vi "sendEmail.vi"(6 "Queue limit":dbl=100.0, 7 "Mail":bool, 8 "error in (no error)":errorcluster, 9 "Recipient's Email Address Address":string="frouman@gmail.com", 10 "Queue Length":dbl, 11 "Acquisition in":refnum<class "Acquisition.lvclass">) -> (0 "error out":errorcluster, 3 "Acquisition out":refnum<class "Acquisition.lvclass">)   [LabVIEW 2014, in "Acquisition.lvclass"]
uses:
  Acquisition.lvclass
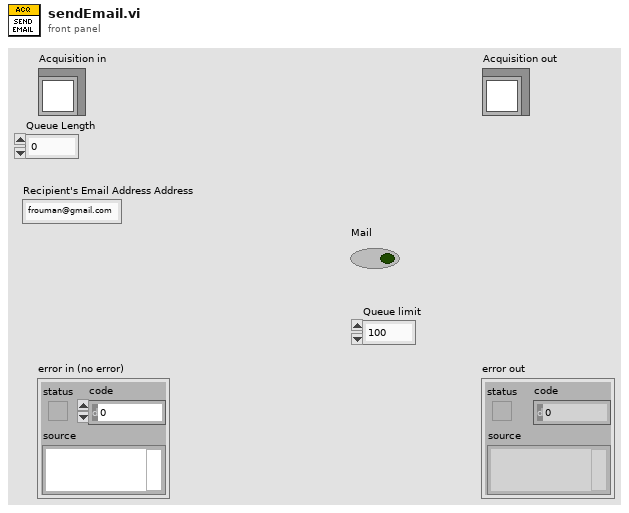
[diagram p1: front panel]
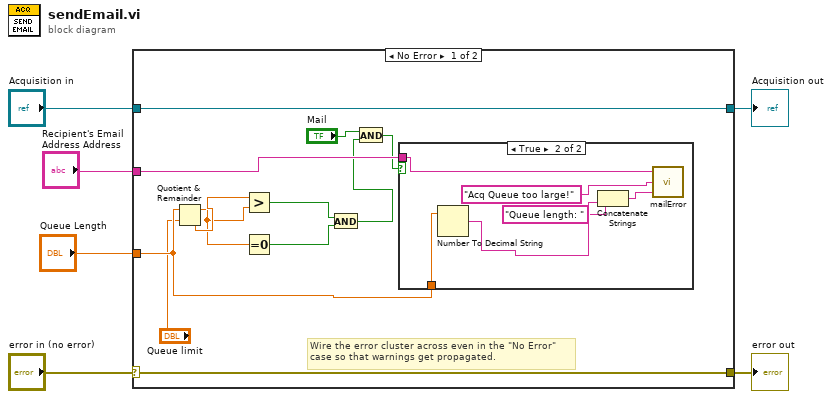
[diagram p0: block diagram]
diagram:
  n1 = case shown="No Error" "error in (no error)" {
    selector: "error in (no error)" -> [w17 w26]
    tunnel: [w17 w26] -> w5
    tunnel: [w18 w25] -> w3
    tunnel: "Acquisition in" -> [w18 w25]
    tunnel: "Queue Length" -> [w12 _]
    tunnel: "Recipient's Email Address Address" -> [w11 _]
    frame No Error {
      # "Wire the error cluster across even in the \"No Error\"\ncase so that warnings get propagated."
      n2 = Quotient & Remainder(x=w12, y="Queue limit") -> (x-y*floor(x/y)=w13:dbl, floor(x/y)=w14:dbl)
      n3 = Greater?(x=w14, y=w13) -> (0:w15:bool)
      n4 = Equal To 0?(x=w13) -> (x = 0?=w16:bool)
      n5 = And(x=w15, y=w16) -> (x .and. y?=w10:bool)
      n6 = And(x="Mail", y=w10) -> (x .and. y?=w8:bool)
      n7 = case shown="True" w8 {
        tunnel: w12 -> [_ w24]
        tunnel: w11 -> [_ w19]
        frame False {
        }
        frame True {
          n8 = Number To Decimal String(number=w24) -> (decimal integer string=w23:string)  [unwired: 1 in]
          n9 = Concatenate Strings("Queue length: " ("string"), w23) -> (w21:string)
          n10 = call "mailError.vi"("Body"=w21, "Subject"="Acq Queue too large!", "Recipient's Email Address Address"=w19) -> ()  [unwired: 1 in]
        }
      }
    }
    frame Error {
    }
  }
  "error out" <- w5
  "Acquisition out" <- w3
